vi "SMC_MoveAbs.vi"(8 "error in (no error)":errorcluster, 9 "WaitUntilReady":bool, 11 "Input Array":dbl[](array[numeric]) format="%.2f") -> (0 "error out":errorcluster)   [LabVIEW 2015]
uses:
  SMC_SubVIs.llb/SMC_ManagerMode.ctl
  SMC_SubVIs.llb/glb_stop.vi
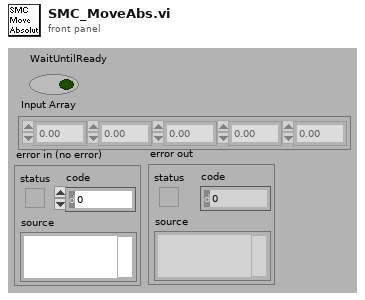
[diagram p1: front panel]
types:
  T1 = typedef "SMC_ManagerMode.ctl" = enum16{"Init", "Get", "SetPosition", "SetStatus", "SetMoving", "SetControllerNr"}
  T2 = typedef "SMC Paras.ctl" = cluster{"VENUS Language":T3, "Number of Axis":u8, "Controller Nr":u8, "Simulation":bool}
  T3 = typedef "VENUSNr.ctl" = enum16{"VENUS 2", "VENUS 1"}
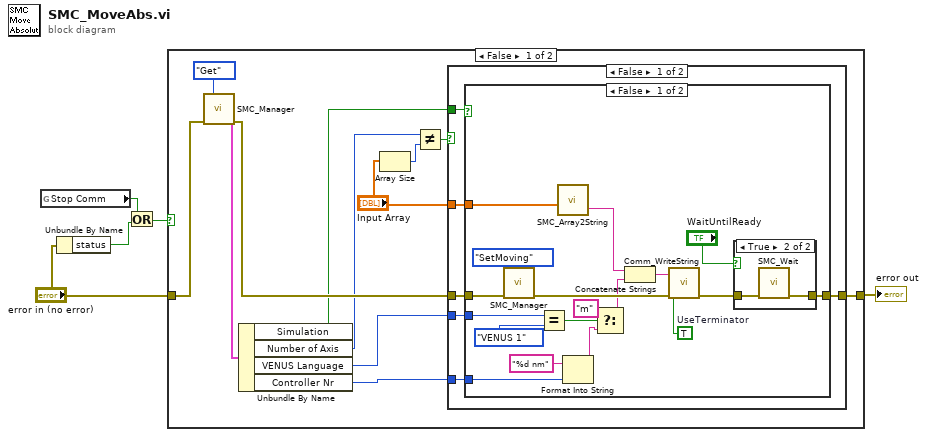
[diagram p0: block diagram]
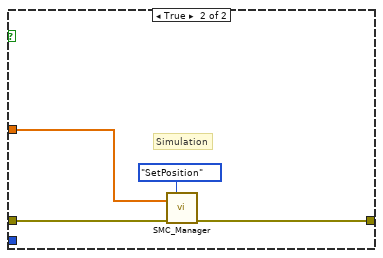
[diagram p3: hidden frame]
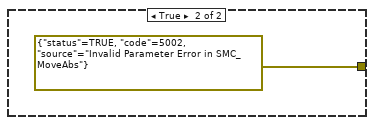
[diagram p4: hidden frame]
diagram:
  n1 = global read "glb_stop.vi" "Stop Comm"() -> (w3:bool)
  n2 = Unbundle By Name("error in (no error)") -> ("status"=w1:bool)
  n3 = Or(x=w3, y=w1) -> (x .or. y?=w2:bool)
  n4 = case shown="False" w2 {
    tunnel: "error in (no error)" -> [w12 w50]
    tunnel: [w13 w50] -> w4
    frame False {
      n5 = call "SMC_Manager.vi"("Mode"=SMC_ManagerMode."Get", "error in (no error)"=w12) -> ("SMC Parameter Out"=w10:T2, "error out"=w11:errorcluster)  [unwired: 9 in, 3 out]
      n6 = Unbundle By Name(w10) -> ("Simulation"=w6:bool, "Number of Axis"=w7:u8, "VENUS Language"=w9:T3, "Controller Nr"=w8:u8)
      n7 = Array Size(array="Input Array") -> (size(s)=w15:i32)
      n8 = Not Equal?(x=w7, y=w15) -> (x != y?=w14:bool)
      n9 = case shown="False" w14 {
        tunnel: "Input Array" -> [w23 _]
        tunnel: [w22 errorcluster {"status"=TRUE, "code"=5002, "source"="Invalid Parameter Error in SMC_MoveAbs"} ("t")] -> w13
        tunnel: w11 -> [w21 _]
        tunnel: w6 -> [w20 _]
        tunnel: w9 -> [w19 _]
        tunnel: w8 -> [w18 _]
        frame False {
          n10 = case shown="False" w20 {
            tunnel: w23 -> [w38 w45]
            tunnel: [w36 w46] -> w22
            tunnel: w21 -> [w40 w47]
            tunnel: w19 -> [w33 _]
            tunnel: w18 -> [w29 _]
            frame False {
              w24 = TRUE  # UseTerminator
              n11 = call "SMC_Manager.vi"("Mode"=SMC_ManagerMode."SetMoving", "error in (no error)"=w40) -> ("error out"=w39:errorcluster)  [unwired: 9 in, 4 out]
              n12 = Equal?(x=w33, y=enum16{"VENUS 2", "VENUS 1"}."VENUS 1") -> (x = y?=w31:bool)
              n13 = call "SMC_Array2String.vi"("Input Array"=w38) -> ("String"=w37:string)  [unwired: 10 in]
              n14 = Format Into String(format string="%d nm" ("Format String"), w29) -> (resulting string=w28:string)  [unwired: 2 in, 1 out]
              n15 = Select(t="m" ("Substring"), s=w31, f=w28) -> (s? t:f=w26:string)
              n16 = Concatenate Strings(w37, w26) -> (w25:string)
              n17 = call "Comm_WriteString.vi"("string to write"=w25, "error in (no error)"=w39, "UseTerminator"=w24) -> ("error out"=w35:errorcluster)  [unwired: 8 in]
              n18 = case shown="True" "WaitUntilReady" {
                tunnel: w35 -> [w42 w44]
                tunnel: [w42 w43] -> w36
                frame False {
                }
                frame True {
                  n19 = call "SMC_Wait.vi"("error in (no error)"=w44) -> ("error out"=w43:errorcluster)  [unwired: 10 in]
                }
              }
            }
            frame True {
              # "Simulation"
              n20 = call "SMC_Manager.vi"("Mode"=SMC_ManagerMode."SetPosition", "PosArraySimu"=w45, "error in (no error)"=w47) -> ("error out"=w46:errorcluster)  [unwired: 8 in, 4 out]
            }
          }
        }
        frame True {
        }
      }
    }
    frame True {
      # "Error, do nothing"
    }
  }
  "error out" <- w4
